vi "Console Example.vi"() -> ()   [LabVIEW 2024, in "serenial-io.ase.console.lvlib"]
uses:
  serenial-io.ase.console.lvlib
  serenial.io-ase/ase/ase.lvclass
  <vilib>/Utility/miscctls.llb/LVPointTypeDef.ctl
  serenial.io-ase/ase/Start Call (Command).vi
panel:
  in  "Write Exit":bool
  in  "Clear Std Out":bool
  in  "Start Console":bool
  in  "Send Terminate":bool
  in  "Clear Std Err":bool
  in  "working directory":path=path "c:/"
  in  "Send":bool
  in  "Cmd":string="echo hello!" caption="Cmd In (can include multiple lines)"
  out "Std Err":string
  out "Std Out":string
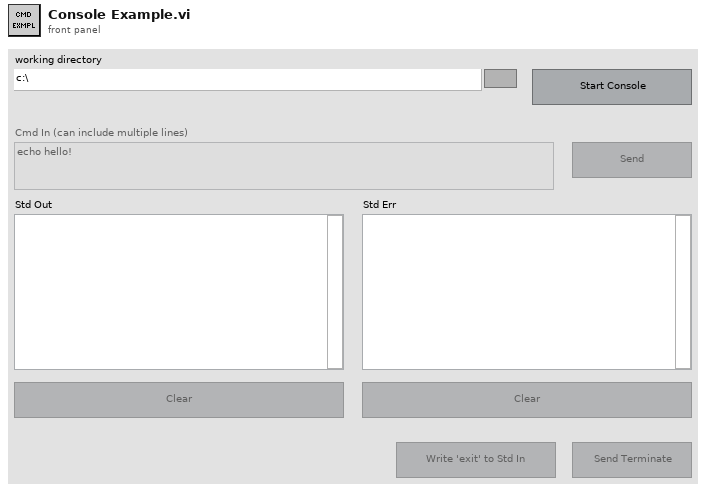
[diagram p1: front panel]
types:
  T1 = enum8{"Enabled", "Disabled", "Disabled and Grayed Out"}
  T2 = typedef "LVPointTypeDef.ctl" = cluster{"Horizontal":i16, "Vertical":i16}
  T3 = typedef "serenial.io-ase.lvlib/ase.lvclass/Event References.ctl" = cluster{"Standard Output":refnum<user-event>, "Standard Error":refnum<user-event>, "Did Exit":refnum<user-event>}
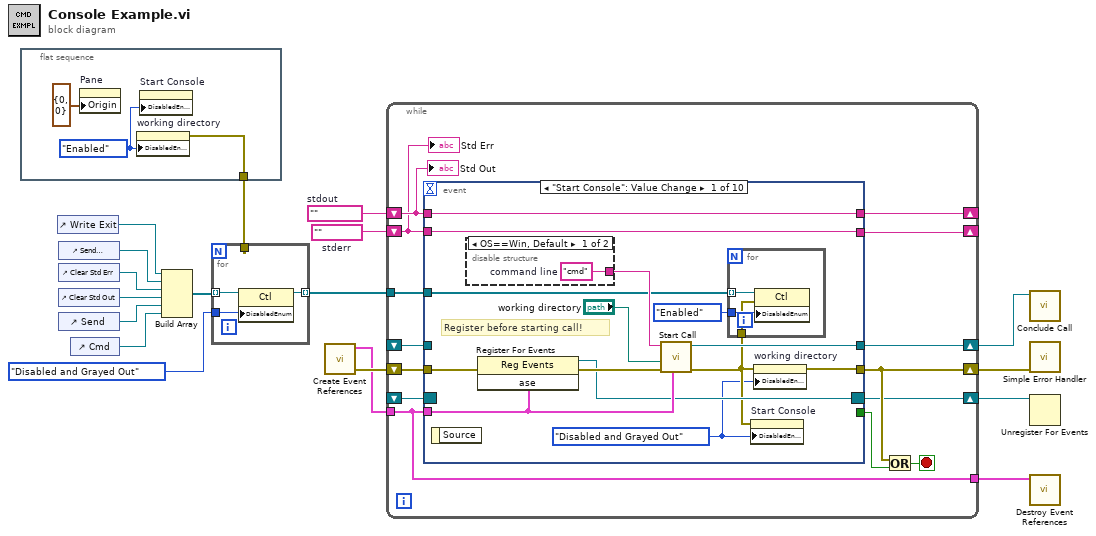
[diagram p0: block diagram]
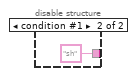
[diagram p2: hidden frame]
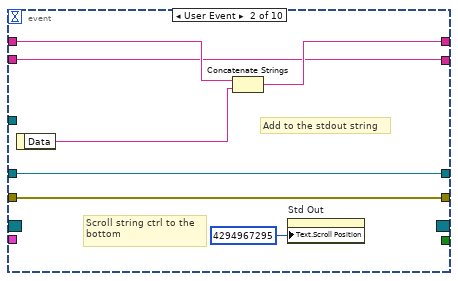
[diagram p3: hidden frame]
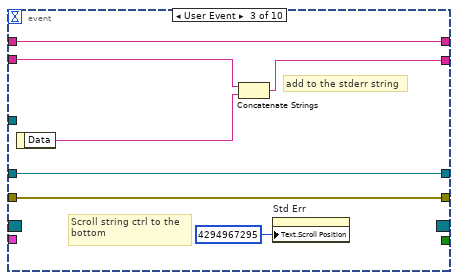
[diagram p4: hidden frame]
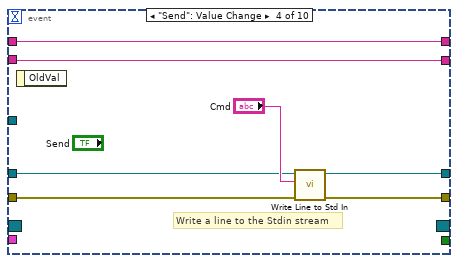
[diagram p5: hidden frame]
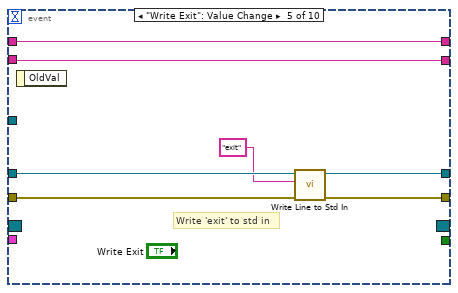
[diagram p6: hidden frame]
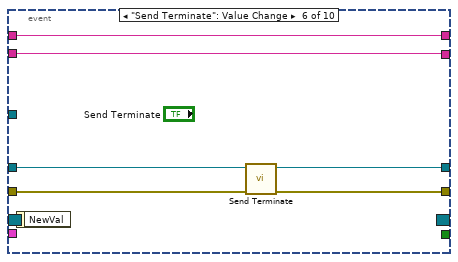
[diagram p7: hidden frame]
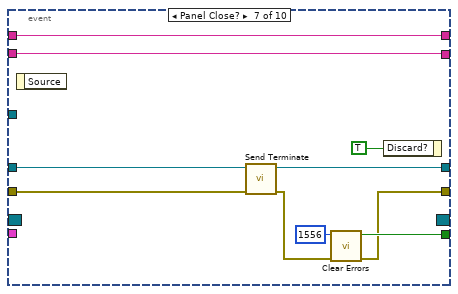
[diagram p8: hidden frame]
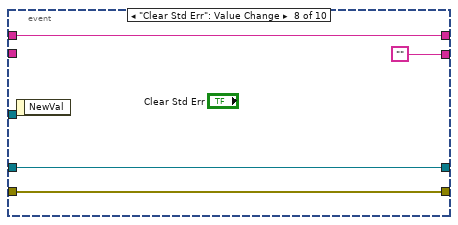
[diagram p9: hidden frame]
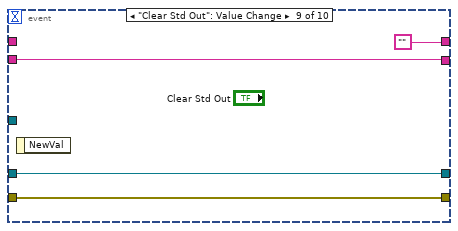
[diagram p10: hidden frame]
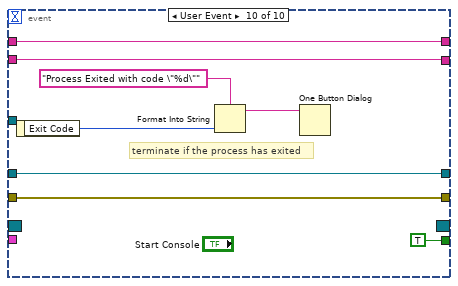
[diagram p11: hidden frame]
diagram:
  w12 = ""  # stderr
  w13 = ""  # stdout
  n1 = flat-sequence {
    tunnel: [w21] -> w3
    frame #0 {
      w19 = T1."Enabled" ("Disabled")
      n2 = property on="Pane" class="Pane"("Origin"=T2 {"Horizontal"=0, "Vertical"=0}) -> ()  [unwired: 2 in, 2 out]
      n3 = property on="working directory" class="Path"("DisabledEnum"=w19) -> (error out=w21:errorcluster)  [unwired: 2 in, 1 out]
      n4 = property on="Start Console" class="Bool"("DisabledEnum"=w19) -> ()  [unwired: 2 in, 2 out]
    }
  }
  n5 = control-ref of="Write Exit"() -> (w2:refnum<vi>)
  n6 = control-ref of="Send Terminate"() -> (w11:refnum<vi>)
  n7 = control-ref of="Clear Std Err"() -> (w10:refnum<vi>)
  n8 = control-ref of="Clear Std Out"() -> (w9:refnum<vi>)
  n9 = control-ref of="Send"() -> (w8:refnum<vi>)
  n10 = control-ref of="Cmd"() -> (w7:refnum<vi>)
  n11 = Build Array(w2, w11, w10, w9, w8, w7) -> (w6:refnum<vi>[])
  n12 = for {
    tunnel: w6 -> [w24] mode=indexing
    tunnel: T1."Disabled and Grayed Out" ("Disabled") -> [w23]
    tunnel: [w22] -> w4 mode=indexing
    tunnel: w3 -> [_]
    n13 = property class="Ctl"(reference=w24, "DisabledEnum"=w23) -> (reference out=w22:refnum<vi>)  [unwired: 1 in, 1 out]
  }
  n14 = call "Create Event References.vi"() -> ("error out"=w18:errorcluster, "ase"=w15:T3)  [unwired: 10 in]
  n15 = while {
    shift-right: [w36] -> w16
    shift-left: _ -> [w35]
    shift-right: [w37] -> w1
    shift-left: w18 -> [w38]
    shift-right: [w33] -> _
    shift-left: w13 -> [w27]
    shift-right: [w30] -> _
    shift-left: w12 -> [w26]
    tunnel: w15 -> [w29]
    tunnel: [w29] -> w14
    shift-right: [w34] -> w17
    shift-left: _ -> [w28]
    tunnel: w4 -> [w25]
    stop <- w31 stop-if-true
    n16 = event shown="[0] \"Start Console\": Value Change" {
      selector: w28 -> [_ _ _ _ _ _ _ _ _ _]
      dyn-events: [w44 _ _ _ _ _ _ _ _ _] -> w34
      timeout: _ -> [_ _ _ _ _ _ _ _ _ _]
      tunnel: [w50 w63 w70 w76 w83 w86 w98 w104 w109 w114] -> w36
      tunnel: w35 -> [_ w63 w70 w72 w80 w87 w99 w104 w109 w114]
      tunnel: w38 -> [w48 w64 w71 w77 w84 w91 w95 w105 w108 w117]
      tunnel: [w41 w64 w71 w78 w85 w90 w92 w105 w108 w117] -> w37
      tunnel: w27 -> [w52 w61 w67 w74 w82 w89 w101 w103 _ w115]
      tunnel: [w52 w62 w67 w74 w82 w89 w101 w103 "" w115] -> w33
      tunnel: [_ _ _ _ _ _ w93 _ _ TRUE] -> w32
      tunnel: w26 -> [w51 w59 w68 w73 w81 w88 w100 _ w107 w116]
      tunnel: [w51 w59 w66 w73 w81 w88 w100 "" w107 w116] -> w30
      tunnel: w29 -> [w46 _ _ _ _ _ _ _ _ _]
      tunnel: w25 -> [w42 _ _ _ _ _ _ _ _ _]
      event "Start Console": Value Change {
        w39 = T1."Disabled and Grayed Out" ("Disabled")
        # "Register before starting call!"
        n17 = event-data() -> ()  [unwired: 1 in, 1 out]
        n18 = disable-structure "Conditional Disable Structure" shown="OS==Win, Default" {
          disable-tunnel: [w56 "sh" ("command line")] -> w49
          frame condition #0 (active) {
            w56 = "cmd"  # command line
          }
          frame condition #1 {
          }
        }
        n19 = register-events(error in=w48, w46) -> (reference out=w44:refnum<event-registration>, error out=w47:errorcluster)  [unwired: 1 in]
        n20 = call-poly "Start Call.vi"("Event References"=w46, "error in"=w47, "Working Directory (default <Not A Path> - System Default)"="working directory", "Command"=w49) -> ("error out"=w40:errorcluster, "New ASE Handle"=w50:refnum<class "ase.lvclass">)  [unwired: 6 in]
        n21 = for {
          tunnel: w42 -> [w55] mode=indexing
          tunnel: T1."Enabled" ("Disabled") -> [w54]
          tunnel: w40 -> [w53]
          n22 = property class="Ctl"(reference=w55, error in=w53, "DisabledEnum"=w54) -> ()  [unwired: 2 out]
        }
        n23 = property on="Start Console" class="Bool"(error in=w40, "DisabledEnum"=w39) -> ()  [unwired: 1 in, 2 out]
        n24 = property on="working directory" class="Path"(error in=w40, "DisabledEnum"=w39) -> (error out=w41:errorcluster)  [unwired: 1 in, 1 out]
      }
      event User Event {
        # "Scroll string ctrl to the \nbottom"
        # "Add to the stdout string"
        n25 = event-data() -> ("Data"=w60:string)  [unwired: 1 in]
        n26 = Concatenate Strings(w61, w60) -> (w62:string)
        n27 = property on="Std Out" class="Str"("Text.Scroll Position"=u32 4294967295) -> ()  [unwired: 2 in, 2 out]
      }
      event User Event {
        # "Scroll string ctrl to the \nbottom"
        # "add to the stderr string"
        n28 = event-data() -> ("Data"=w69:string)  [unwired: 1 in]
        n29 = Concatenate Strings(w68, w69) -> (w66:string)
        n30 = property on="Std Err" class="Str"("Text.Scroll Position"=u32 4294967295) -> ()  [unwired: 2 in, 2 out]
      }
      event "Send": Value Change {
        # "Write a line to the Stdin stream"
        n31 = event-data() -> ()  [unwired: 1 in, 1 out]
        n32 = call "Write Line to Std In .vi"("error in"=w77, "Input"="Cmd", "ASE Handle"=w72) -> ("error out"=w78:errorcluster, "ASE Handle Duplicate"=w76:refnum<class "ase.lvclass">)  [unwired: 6 in, 1 out]
      }
      event "Write Exit": Value Change {
        # "Write 'exit' to std in"
        n33 = event-data() -> ()  [unwired: 1 in, 1 out]
        n34 = call "Write Line to Std In .vi"("error in"=w84, "Input"="exit", "ASE Handle"=w80) -> ("error out"=w85:errorcluster, "ASE Handle Duplicate"=w83:refnum<class "ase.lvclass">)  [unwired: 6 in, 1 out]
      }
      event "Send Terminate": Value Change {
        n35 = event-data() -> ()  [unwired: 1 in, 1 out]
        n36 = call "Send Terminate.vi"("error in"=w91, "ASE Handle"=w87) -> ("error out"=w90:errorcluster, "ASE Handle Duplicate"=w86:refnum<class "ase.lvclass">)  [unwired: 7 in, 1 out]
      }
      event Panel Close? {
        n37 = event-data() -> ()  [unwired: 1 in, 1 out]
        n38 = call "Send Terminate.vi"("error in"=w95, "ASE Handle"=w99) -> ("error out"=w96:errorcluster, "ASE Handle Duplicate"=w98:refnum<class "ase.lvclass">)  [unwired: 7 in, 1 out]
        n39 = call <vilib>:"Clear Errors.vi"("error in (no error)"=w96, "specific error code to clear (0: all)"=1556) -> ("error out"=w92:errorcluster, "specific error cleared?"=w93:bool)  [unwired: 4 in]
        n40 = event-data("Discard?"=TRUE) -> ()  [unwired: 1 in, 1 out]
      }
      event "Clear Std Err": Value Change {
        n41 = event-data() -> ()  [unwired: 1 in, 1 out]
      }
      event "Clear Std Out": Value Change {
        n42 = event-data() -> ()  [unwired: 1 in, 1 out]
      }
      event User Event {
        # "terminate if the process has exited"
        n43 = event-data() -> ("Exit Code"=w112:i32)  [unwired: 1 in]
        n44 = Format Into String(format string="Process Exited with code \"%d\"", w112) -> (resulting string=w111:string)  [unwired: 2 in, 1 out]
        n45 = One Button Dialog(message=w111) -> ()  [unwired: 1 in, 1 out]
      }
    }
    n46 = Or(x=w37, y=w32) -> (x .or. y?=w31:bool)
    "Std Err" <- w26
    "Std Out" <- w27
  }
  n47 = call "Conclude Call.vi"("ASE Handle"=w16) -> ()  [unwired: 8 in, 3 out]
  n48 = call <vilib>:"Simple Error Handler.vi"("error in (no error)"=w1) -> ()  [unwired: 4 in, 5 out]
  n49 = Unregister For Events(event registration refnum=w17) -> ()  [unwired: 1 in, 1 out]
  n50 = call "Destroy Event References.vi"("Event References"=w14) -> ()  [unwired: 10 in, 1 out]
